vi "LS 340 set T.vi"(0 "Set point":dbl format="%.2f", 1 "GPIB Adress":i16) -> ()   [LabVIEW 2015]
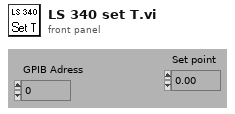
[diagram p1: front panel]
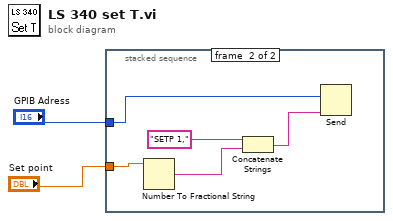
[diagram p0: block diagram]
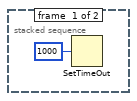
[diagram p2: hidden frame]
diagram:
  n1 = stacked-sequence {
    tunnel: "GPIB Adress" -> [_ w8]
    tunnel: "Set point" -> [_ w5]
    frame #0 {
      n2 = SetTimeOut(1:1000 ("new timeout (10000)")) -> ()  [unwired: 1 out]
    }
    frame #1 {
      n3 = Number To Fractional String(number=w5) -> (F-format string=w7:string)  [unwired: 3 in]
      n4 = Concatenate Strings("SETP 1," ("data string"), w7) -> (w4:string)
      n5 = Send(2:w8, 5:w4) -> ()  [unwired: 3 in, 3 out]
    }
  }
